vi "Pass if Test Run Result Count.vi"(8 "error in (no error)":errorcluster, 9 "timeout in ms (0)":i32, 10 "Required Number of Suite Results":i32, 11 "Test Runner Test in":refnum<class "Test Runner Test.lvclass">) -> (0 "error out":errorcluster, 3 "Test Runner Test out":refnum<class "Test Runner Test.lvclass">)   [LabVIEW 2020, in "Test Runner Test.lvclass"]
uses:
  Test Runner Test.lvclass
  C:/Program Files (x86)/National Instruments/LabVIEW 2020/vi.lib/Astemes/LUnit/Test Case.lvclass
  source/Core/Result/Result.ctl
  source/Core/Result/Status.ctl
  source/Core/Result/Type.ctl
  Test Runner Test.lvclass/Test Runner Test.ctl
  <vilib>/Astemes/LUnit/Test Case.lvclass/Test Case.ctl
  8cc7373c-284c-4d8b-bf42-1ac05e0709c9.vi
  <vilib>/Astemes/LUnit/Palette/Pass.vi
  <vilib>/Astemes/LUnit/Palette/Fail.vi
  <vilib>/Astemes/LUnit/Compare Variants.vi
  <vilib>/Astemes/LUnit/Describe Comparison.vi
  <vilib>/Astemes/LUnit/Set Assertion Type.vi
  <vilib>/Astemes/LUnit/Add test result.vi
  <vilib>/Astemes/LUnit/Variant to string.vi
  <vilib>/Astemes/LUnit/LUnit Record Assertion Result.vi
  <vilib>/Astemes/LUnit/LUnit Aggregate Assertion Results.vi
  <vilib>/Astemes/LUnit/Method Result/LUnit Merge Status.vi
  <vilib>/Astemes/LUnit/LUnit Concatenate result strings.vi
  <vilib>/Utility/Data Type/Get Type Information.vi
  <vilib>/Utility/LVClass/Get LV Class Name.vi
  source/Core/Result/Result.lvlib
panel:
  out "Array":T1[](array[typedef])
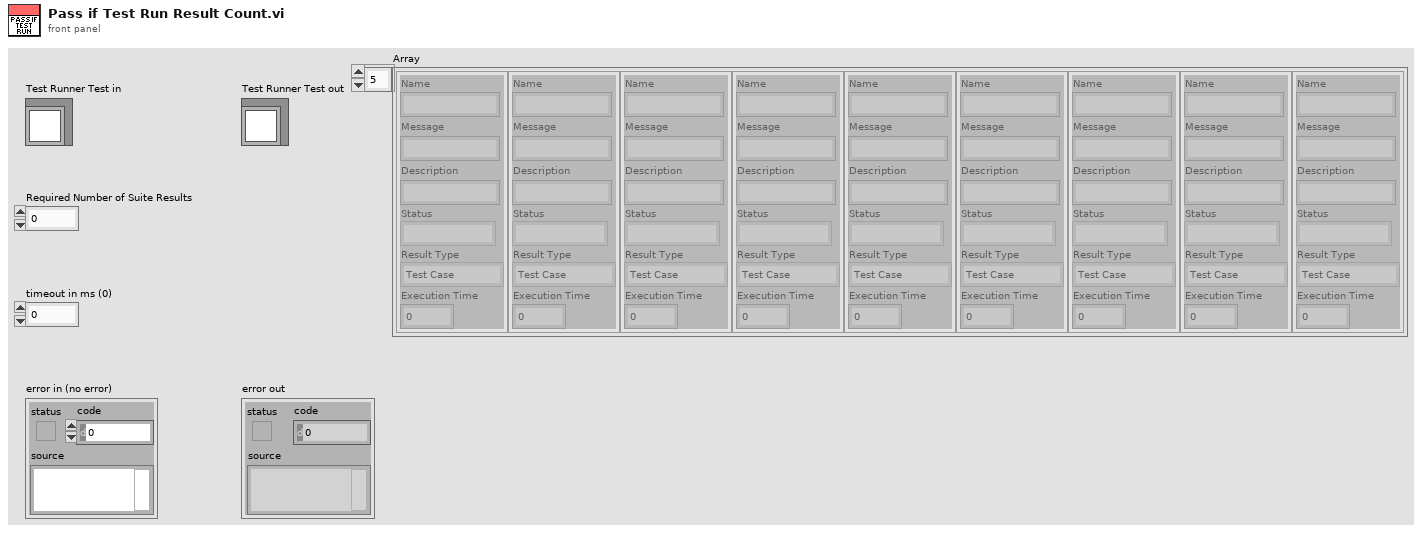
[diagram p1: front panel]
types:
  T1 = typedef "Result.lvlib/Result.ctl" = cluster{"Name":string, "Message":string, "Description":string, "Status":T2, "Result Type":T3, "Execution Time":dbl}
  T2 = typedef "Result.lvlib/Status.ctl" = enum16{"", "Passed", "Failed", "Error", "Skipped", "Setup Error", "Broken", "Teardown Error"}
  T3 = typedef "Result.lvlib/Type.ctl" = enum16{"Test Case", "Test Suite", "Test Run", "Pass", "Fail", "Skip", "Pass if", "Fail if", "Pass if Error", "Fail if Error", "Pass if Equal", "Fail if Equal"}
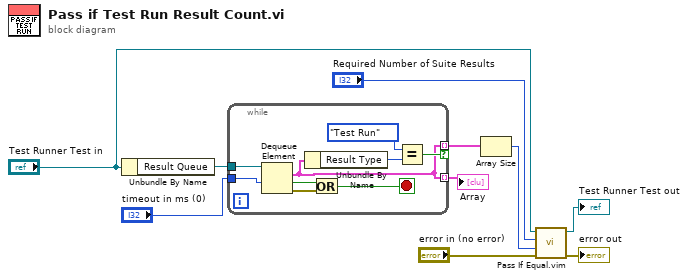
[diagram p0: block diagram]
diagram:
  n1 = Unbundle By Name("Test Runner Test in") -> ("Result Queue"=w6:refnum<queue>)
  n2 = while {
    tunnel: w6 -> [w19]
    tunnel: "timeout in ms (0)" -> [w18]
    tunnel: [w11] -> w4 mode=indexing if=w15
    tunnel: [w11] -> w1 mode=indexing
    stop <- w13 stop-if-true
    n3 = Dequeue Element(queue=w19, timeout in ms (-1)=w18) -> (element=w11:T1, timed out?=w14:bool, error out=w12:errorcluster)  [unwired: 1 in, 1 out]
    n4 = Unbundle By Name(w11) -> ("Result Type"=w17:T3)
    n5 = Or(x=w14, y=w12) -> (x .or. y?=w13:bool)
    n6 = Equal?(x=Type."Test Run", y=w17) -> (x = y?=w15:bool)
  }
  "Array" <- w1
  n7 = Array Size(array=w4) -> (size(s)=w2:i32)
  n8 = call "Pass If Equal.vim"("error in (no error)"="error in (no error)", "Actual"=w2, "Expected"="Required Number of Suite Results", "LUnit Test Case In"="Test Runner Test in") -> ("error out"=→"error out":errorcluster, "LUnit Test Case Out"=→"Test Runner Test out":refnum<class "Test Runner Test.lvclass">)  [unwired: 6 in]
